vi "Async Start recording video from CamServer.vi"(1 "Quality":i32=750 min=0 max=1000, 2 "Resolution":T1=1 items=["Low", "Med.", "High", "Max."], 3 "Camera":T2="Travcam") -> (0 "Error out":errorcluster)   [LabVIEW 2015]
doc: "Asynchronously starts recording video from the selected camera on the camera server. The user must subsequently run the \"Async Stop and get video....\" vi to end the recording and save the video file."
uses:
  Camera enum/Camera enum.ctl
  Camera enum/Camera resolution.ctl
panel:
  # "PN 21/08/15"
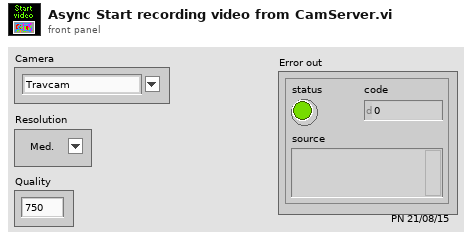
[diagram p1: front panel]
types:
  T1 = typedef "Camera resolution.ctl" = u8
  T2 = typedef "Camera enum.ctl" = string
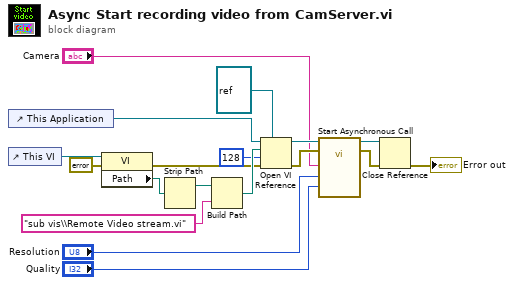
[diagram p0: block diagram]
diagram:
  n1 = control-ref of="This Application"() -> (w13:refnum<vi>)
  n2 = control-ref of="This VI"() -> (w18:refnum<vi>)
  n3 = property class="VI"(reference=w18, error in=errorcluster {"status"=FALSE, "code"=0, "source"=""} ("error in (no error)")) -> (error out=w15:errorcluster, "Path"=w11:path)  [unwired: 1 out]
  n4 = Strip Path(path=w11) -> (stripped path=w10:path)  [unwired: 1 out]
  n5 = Build Path(base path=w10, name or relative path="sub vis\\Remote Video stream.vi") -> (appended path=w16:path)
  n6 = Open VI Reference(type specifier VI Refnum (for type only)=refnum<vi> refnum, application reference (local)=w13, vi path=w16, options=128, error in (no error)=w15) -> (vi reference=w9:refnum<vi>, error out=w8:errorcluster)  [unwired: 1 in]
  n7 = call-by-ref "Start Asynchronous Call"(reference=w9, error in=w8, "Quality"="Quality", "Resolution"="Resolution", "Camera"="Camera") -> (reference out=w5:refnum<vi>, error out=w4:errorcluster)  [unwired: 1 out]
  n8 = Close Reference(reference=w5, error in (no error)=w4) -> (error out=→"Error out":errorcluster)
